vi "PD 120VAC.vi"(3 "120 VAC":bool=TRUE, 8 "error in":errorcluster) -> (0 "error out":errorcluster)   [LabVIEW 2022 SP3]
uses:
  <vilib>/DAQmx/write.llb/DAQmx Write (Digital Bool 1Line 1Point).vi
  <vilib>/DAQmx/miscellaneous.llb/DAQmx Fill In Error Info.vi
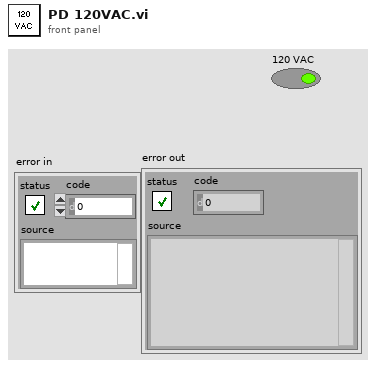
[diagram p1: front panel]
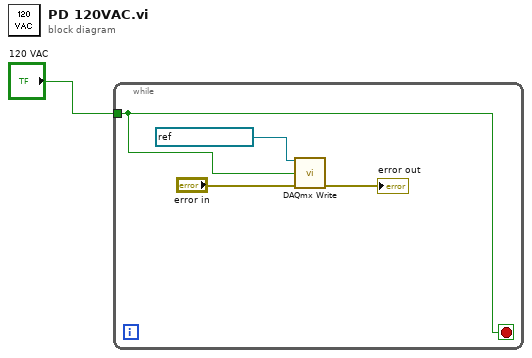
[diagram p0: block diagram]
diagram:
  n1 = while {
    tunnel: "120 VAC" -> [w2]
    stop <- w2 stop-if-true
    n2 = call-poly <vilib>:"DAQmx Write.vi"("task/channels in"=refnum<k21> "FTS2_120VAC", "data"=w2, "error in"="error in") -> ("error out"=→"error out":errorcluster)  [unwired: 10 in, 2 out]
  }
